vi "Write Limits.vi"(8 "error in":errorcluster, 10 "Limits":T1, 11 "PowerSupply in":refnum<class "PowerSupply.lvclass">) -> (0 "error out":errorcluster, 3 "PowerSupply out":refnum<class "PowerSupply.lvclass">)   [LabVIEW 2019, in "PowerSupply.lvlib" / "PowerSupply.lvclass"]
uses:
  Library/PowerSupply.lvclass
  Custom Controls/Limits.ctl
  Library/PowerSupply.lvclass/PowerSupply.ctl
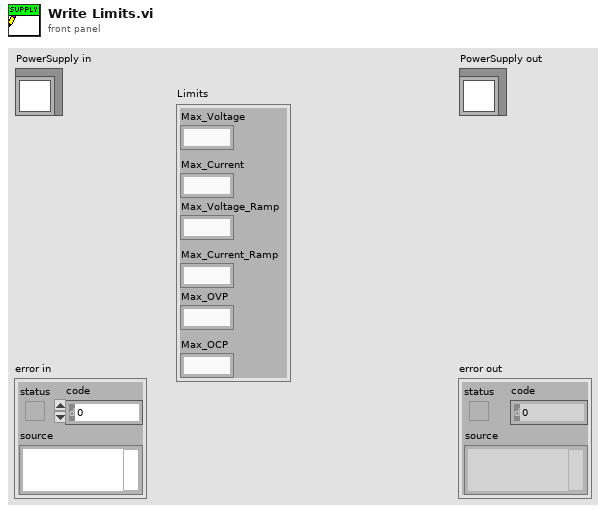
[diagram p1: front panel]
types:
  T1 = typedef "PowerSupply.lvlib/PowerSupply.lvclass/Limits.ctl" = cluster{"Max_Current":dbl, "Max_Voltage":dbl, "Max_Current_Ramp":dbl, "Max_Voltage_Ramp":dbl, "Max_OCP":dbl, "Max_OVP":dbl}
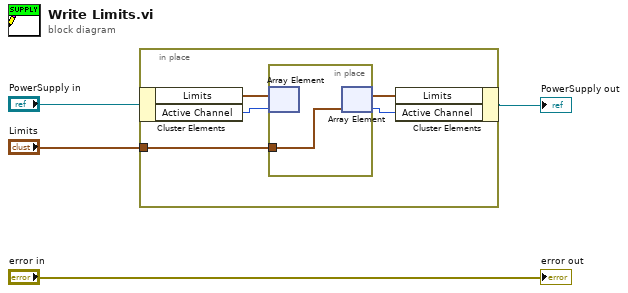
[diagram p0: block diagram]
diagram:
  n1 = in-place {
    in-place-border: "Limits" -> [w5]
    n2 = in-place-cluster #1("PowerSupply in") -> ("Limits"=w9:T1[], "Active Channel"=w8:u32)
    n3 = in-place {
      in-place-border: w5 -> [w10]
      n4 = in-place-array #2(w9, w8) -> ()  [unwired: 1 out]
      n5 = in-place-array #2(w10) -> (w7:T1[], w6:i32)
    }
    n6 = in-place-cluster #1("Limits"=w7, "Active Channel"=w6) -> (→"PowerSupply out":refnum<class "PowerSupply.lvclass">)
  }
  "error out" <- "error in"
